vi "Mode to string.vi"(11 "Mode":T1) -> (3 "String":string)   [LabVIEW 2019, in "STAV lib.lvlib"]
uses:
  STAV lib.lvlib
  Param Mode.ctl
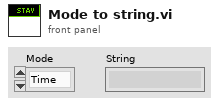
[diagram p1: front panel]
types:
  T1 = typedef "STAV lib.lvlib/Param Mode.ctl" = enum16{"Time", "Cycles"}
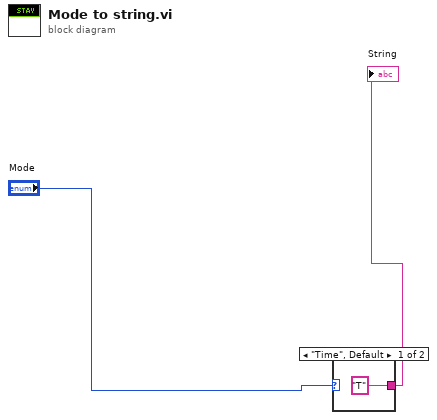
[diagram p0: block diagram]
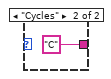
[diagram p2: hidden frame]
diagram:
  n1 = case shown="\"Time\", Default" "Mode" {
    tunnel: ["T" "C"] -> w2
    frame "Time", Default {
    }
    frame "Cycles" {
    }
  }
  "String" <- w2
